vi "SubVI_StopJoystickDrift_TeleOp.vi"(11 "upper limit in":dbl) -> (3 "upper limit out":dbl)   [LabVIEW 2017]
doc: "this sub VI intakes joystick values and eliminates drift and jamming near zero (.25)"
uses:
  <vilib>/gmath/NI_Gmath.lvlib
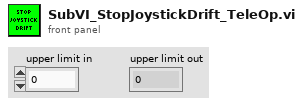
[diagram p1: front panel]
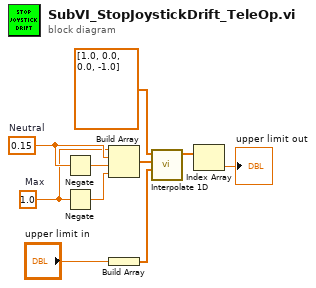
[diagram p0: block diagram]
diagram:
  w6 = 0.15  # Neutral
  w5 = 1.0  # Max
  n1 = Negate(x=w6) -> (-x=w3:dbl)
  n2 = Negate(x=w5) -> (-x=w4:dbl)
  n3 = Build Array(w5, w6, w3, w4) -> (w8:dbl[])
  n4 = Build Array("upper limit in") -> (w10:dbl[])
  n5 = call <vilib>:"Interpolate 1D.vi"("xi"=w10, "X"=w8, "Y"=dbl[] [1.0, 0.0, 0.0, -1.0] ("X")) -> ("yi"=w9:dbl[])  [unwired: 6 in, 2 out]
  n6 = Index Array(array=w9) -> (element=→"upper limit out":dbl)  [unwired: 1 in]
